vi "MaxEye_ATE_New_Load Configuration_Load_from_File.vi"(0 "file path (use dialog)":path, 5 "Variant In":variant, 7 "Config Header":string, 11 "error in (no error)":errorcluster) -> (4 "Variant Out":variant, 15 "error out":errorcluster)   [LabVIEW 2021]
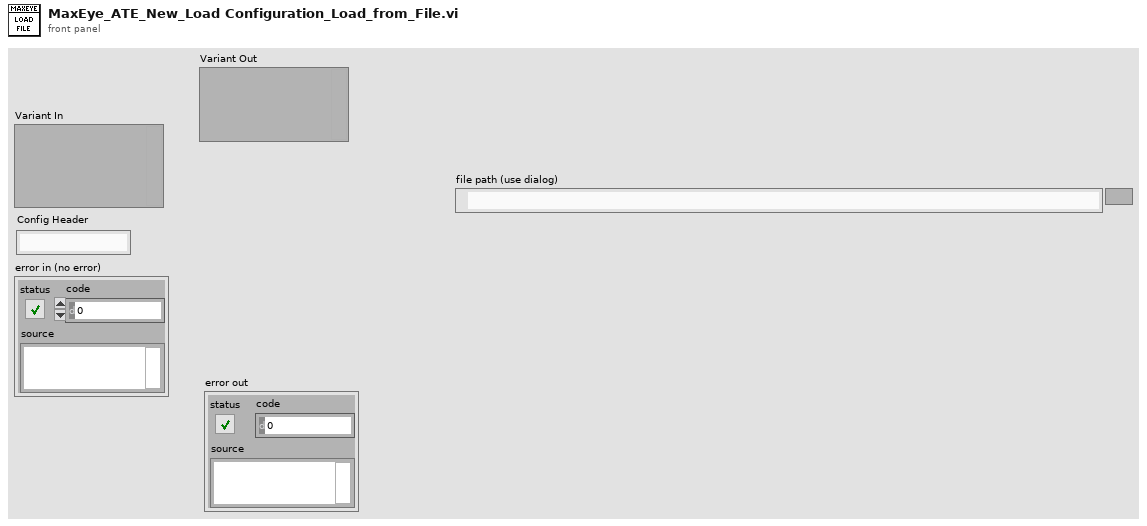
[diagram p1: front panel]
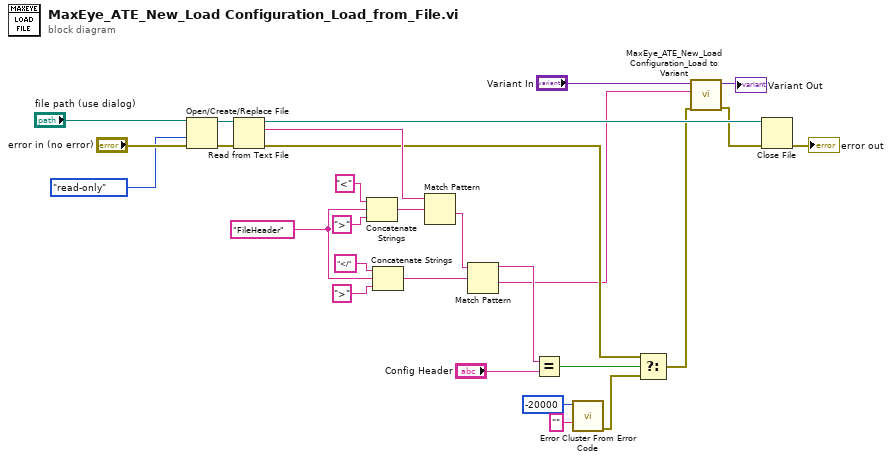
[diagram p0: block diagram]
diagram:
  w15 = "FileHeader" ("string")
  n1 = Open/Create/Replace File(file path (use dialog)="file path (use dialog)", error in="error in (no error)", access (0:read/write)=enum16{"read/write", "read-only", "write-only"}."read-only") -> (refnum out=w24:refnum<file>, error out=w25:errorcluster)  [unwired: 3 in, 1 out]
  n2 = Read from Text File(file (use dialog)=w24, error in=w25) -> (refnum out=w23:refnum<file>, text=w12:string, error out=w10:errorcluster)  [unwired: 2 in, 1 out]
  n3 = Concatenate Strings("<" ("string"), w15, ">" ("string")) -> (w16:string)
  n4 = Concatenate Strings("</" ("string"), w15, ">" ("string")) -> (w17:string)
  n5 = Match Pattern(string=w12, regular expression=w16) -> (after substring=w22:string)  [unwired: 1 in, 3 out]
  n6 = Match Pattern(string=w22, regular expression=w17) -> (before substring=w14:string, after substring=w3:string)  [unwired: 1 in, 2 out]
  n7 = Equal?(x=w14, y="Config Header") -> (x = y?=w11:bool)
  n8 = call <vilib>:"Error Cluster From Error Code.vi"("error message (\"\")"="" ("error message (\"\")"), "error code (0)"=-20000) -> ("error out"=w9:errorcluster)  [unwired: 7 in]
  n9 = Select(t=w10, s=w11, f=w9) -> (s? t:f=w2:errorcluster)
  n10 = call "MaxEye_ATE_New_Load Configuration_Load to Variant.vi"("error in (no error)"=w2, "File Data"=w3, "Variant In"="Variant In") -> ("error out"=w1:errorcluster, "Variant Out"=→"Variant Out":variant)  [unwired: 7 in]
  n11 = Close File(refnum=w23, error in=w1) -> (error out=→"error out":errorcluster)  [unwired: 1 out]
